vi "sortByChannelNumber.vi"(8 "error in (no error)":errorcluster, 10 "data in":T1(array[cluster]), 11 "DeviceData in":refnum<class "DeviceData.lvclass">) -> (0 "error out":errorcluster, 2 "data out":T1(array[cluster]), 3 "DeviceData out":refnum<class "DeviceData.lvclass">)   [LabVIEW 2009, in "DataMappers.lvlib" / "DeviceData.lvclass"]
uses:
  DeviceData.lvclass
  DatabaseHelpers/Database Objects/Channel/Channel.lvclass
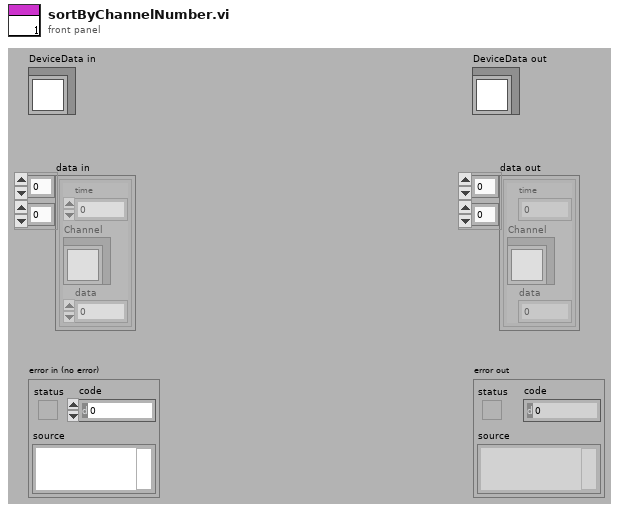
[diagram p1: front panel]
types:
  T1 = cluster{"time":dbl, "Channel":refnum<class "Channel.lvclass">, "data":dbl}[][]
  T2 = cluster{"time":dbl, "Channel":refnum<class "Channel.lvclass">, "data":dbl}
  T3 = cluster{"time":dbl, "Channel":refnum<class "Channel.lvclass">, "data":dbl}[]
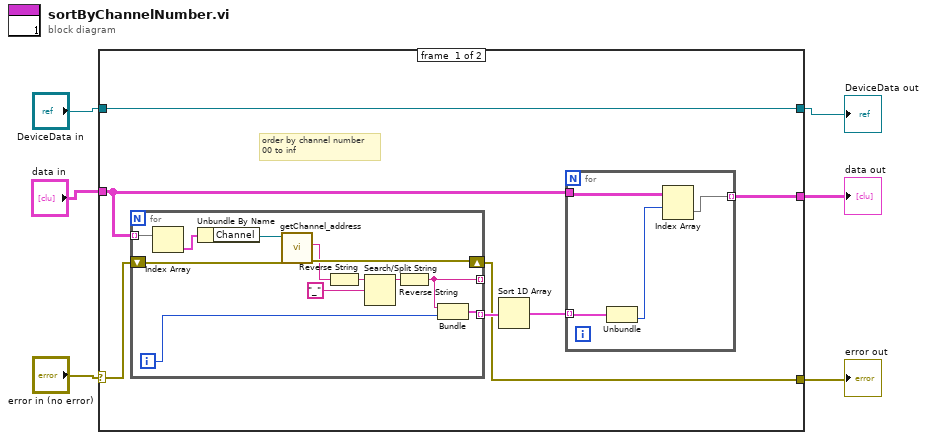
[diagram p0: block diagram]
diagram:
  n1 = case shown="No Error" "error in (no error)" {
    selector: "error in (no error)" -> [w8 w31]
    tunnel: [w7 w31] -> w2
    tunnel: [w13 w30] -> w1
    tunnel: "DeviceData in" -> [w13 w30]
    tunnel: "data in" -> [w10 _]
    tunnel: [w9 _] -> w4
    frame #0 {
      # "order by channel number\n00 to inf"
      n2 = for {
        tunnel: [w20] -> _ mode=indexing
        tunnel: w10 -> [w22] mode=indexing
        shift-right: [w27] -> w7
        shift-left: w8 -> [w28]
        tunnel: [w18] -> w12 mode=indexing
        i -> [w19]
        n3 = Index Array(array=w22) -> (element=w21:T2)  [unwired: 1 in]
        n4 = Unbundle By Name(w21) -> ("Channel"=w29:refnum<class "Channel.lvclass">)
        n5 = call "getChannel_address.vi"("error in (no error)"=w28, "Channel.lvclass in"=w29) -> ("error out"=w27:errorcluster, "channel_address"=w26:string)  [unwired: 7 in, 1 out]
        n6 = Reverse String(1:w26) -> (0:w24:string)
        n7 = Search/Split String(string=w24, search string/char (-)="_") -> (substring before match=w23:string)  [unwired: 1 in, 2 out]
        n8 = Reverse String(1:w23) -> (0:w20:string)
        n9 = Bundle(w20, w19) -> (w18:cluster{string, i32})  [unwired: 1 in]
      }
      n10 = Sort 1D Array(array=w12) -> (sorted array=w11:cluster{string, i32}[])
      n11 = for {
        tunnel: w11 -> [w17] mode=indexing
        tunnel: w10 -> [w15]
        tunnel: [w14] -> w9 mode=indexing
        n12 = Unbundle(w17) -> (w16:i32)  [unwired: 1 out]
        n13 = Index Array(array=w15, index (row)=w16) -> (element=w14:T3)  [unwired: 1 in]
      }
    }
    frame #1 {
    }
  }
  "error out" <- w2
  "DeviceData out" <- w1
  "data out" <- w4
